vi "Read Element.vi"(8 "error in (no error)":errorcluster, 11 "Const_WFM in":refnum<class "Const_WFM.lvclass">) -> (0 "error out":errorcluster, 2 "Element":dbl, 3 "Const_WFM out":refnum<class "Const_WFM.lvclass">)   [LabVIEW 2021, in "Const_WFM.lvclass"]
uses:
  Const_WFM.lvclass
  Const_WFM.lvclass/Const_WFM.ctl
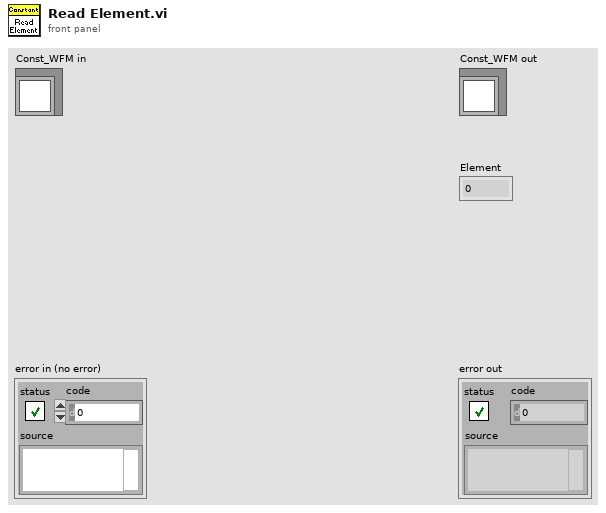
[diagram p1: front panel]
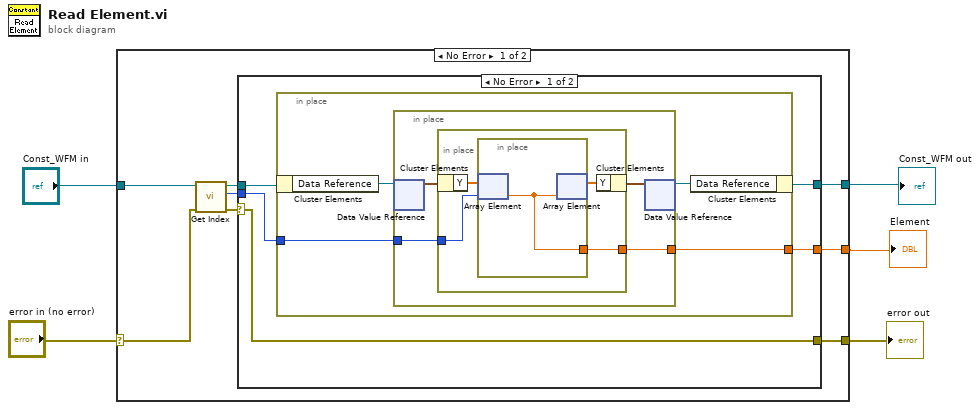
[diagram p0: block diagram]
diagram:
  n1 = case shown="No Error" "error in (no error)" {
    selector: "error in (no error)" -> [w8 w34]
    tunnel: "Const_WFM in" -> [w11 w35]
    tunnel: [w13 w35] -> w5
    tunnel: [w12 _] -> w1
    tunnel: [w6 w34] -> w2
    frame No Error {
      n2 = call-dynamic "Get Index.vi"("error in (no error)"=w8, "Abs_Waveform in"=w11) -> ("error out"=w7:errorcluster, "Index"=w9:i32, "Abs_Waveform out"=w10:refnum<class "Const_WFM.lvclass">)  [unwired: 7 in]
      n3 = case shown="No Error" w7 {
        selector: w7 -> [w14 w33]
        tunnel: [w18 w32] -> w13
        tunnel: [w17 _] -> w12
        tunnel: w10 -> [w16 w32]
        tunnel: w9 -> [w15 _]
        tunnel: [w14 w33] -> w6
        frame No Error {
          n4 = in-place {
            in-place-border: [w20] -> w17
            in-place-border: w15 -> [w19]
            n5 = in-place-cluster #1(w16) -> ("Data Reference"=w22:refnum<data-value>)
            n6 = in-place {
              in-place-border: [w24] -> w20
              in-place-border: w19 -> [w23]
              n7 = in-place-dvr #2(w22) -> (w26:waveform(dbl))  [unwired: 1 out]
              n8 = in-place {
                in-place-border: [w28] -> w24
                in-place-border: w23 -> [w27]
                n9 = in-place-cluster #3(w26) -> ("Y"=w30:dbl[])
                n10 = in-place {
                  in-place-border: [w31] -> w28
                  n11 = in-place-array #4(w30, w27) -> (w31:dbl)
                  n12 = in-place-array #4(w31) -> (w29:dbl[])  [unwired: 1 out]
                }
                n13 = in-place-cluster #3("Y"=w29) -> (w25:waveform(dbl))
              }
              n14 = in-place-dvr #2(w25) -> (w21:refnum<data-value>)  [unwired: 1 out]
            }
            n15 = in-place-cluster #1("Data Reference"=w21) -> (w18:refnum<class "Const_WFM.lvclass">)
          }
        }
        frame Error {
        }
      }
    }
    frame Error {
    }
  }
  "error out" <- w2
  "Const_WFM out" <- w5
  "Element" <- w1
